vi "RemoteForOldJoystick.vi"() -> ()   [LabVIEW 2020]
uses:
  oldStudicaJoystick.ctl
  <vilib>/Platform/TimedLoop/XDataNode/timing_clust.ctl
  <vilib>/Platform/TimedLoop/XDataNode/nitl_modes.ctl
  <vilib>/Platform/TimedLoop/XDataNode/wakeup.ctl
  <vilib>/CISH Robotics/L4VMX TitanQuad/Motor ID.ctl
  <vilib>/CISH Robotics/L4VMX VMXpi/Type Def/VMX Channel Index.ctl
  <vilib>/CISH Robotics/L4VMX TitanQuad/TitanQuad.lvclass
  <vilib>/platform/TimedLoop/XDataNode/XDataNode.xnode
  <vilib>/ReMiSYS Technology/RemoteToolkit/Receiver/Receiver.lvclass
  <vilib>/CISH Robotics/L4VMX VMXpi/L4VMX.lvlib
  <vilib>/CISH Robotics/L4VMX VMXpi/Digital Input/Digital Input.lvclass
  <vilib>/Platform/TimedLoop/XDataNode/XDNodeRunTimeDep.lvlib
panel:
  in  "turnSpeed":dbl=100.0
  in  "reset Encoder":bool
  out "Finished Late? [i-1]":bool
  in  "error in (no error)":errorcluster
  out "Enc [M0, M1, M2] (deg)":dbl[](array[numeric])
  out "error out":errorcluster
  out "StudicaJoystick":T1
  out "Stop0":bool
  out "Error Out":errorcluster
  in  "Stop":bool
  out "Received?":bool
  # "61 * 16"
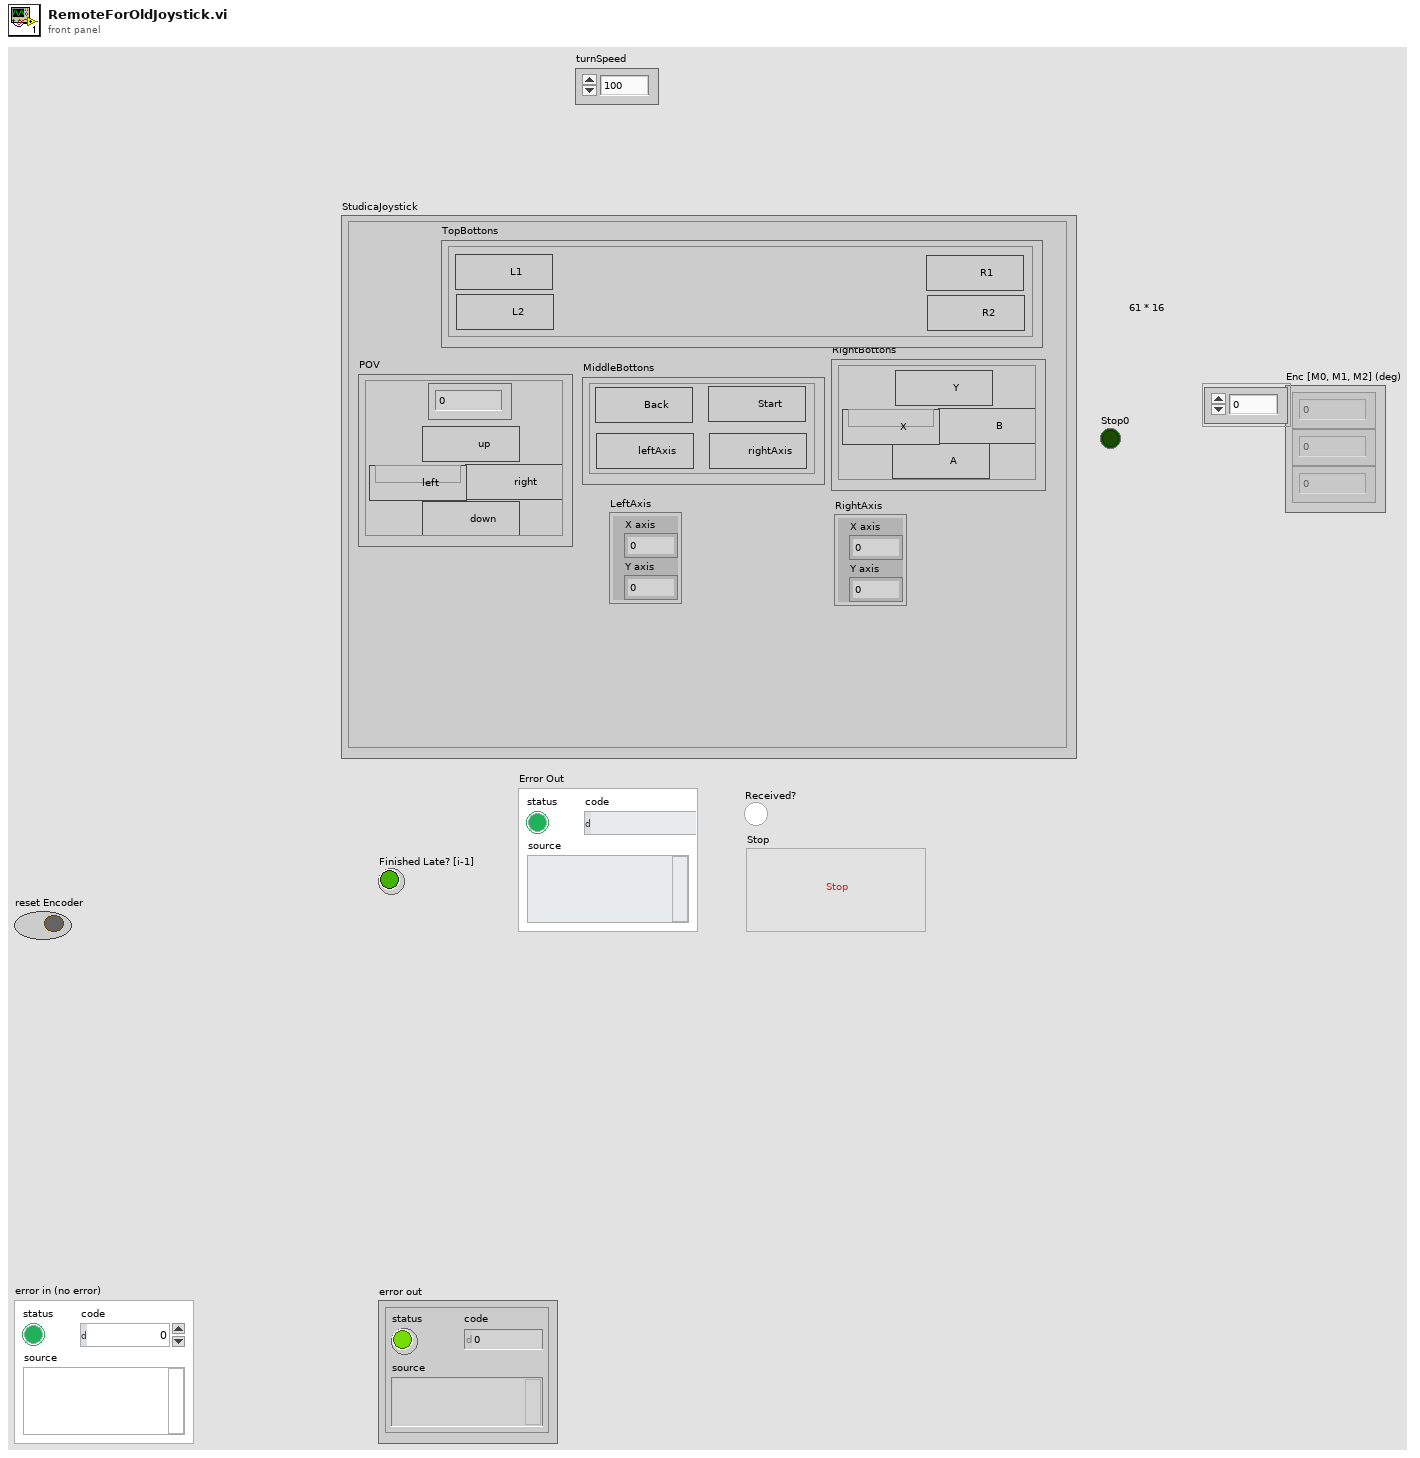
[diagram p1: front panel]
types:
  T1 = typedef "oldStudicaJoystick.ctl" = cluster{"LeftAxis":cluster{"X axis":i32, "Y axis":i32}, "RightAxis":cluster{"X axis":i32, "Y axis":i32}, "RightBottons":cluster{"A":bool, "B":bool, "X":bool, "Y":bool}, "TopBottons":cluster{"Left1":bool, "Left2":bool, "Right1":bool, "Right2":bool}, "MiddleBottons":cluster{"Back":bool, "Play Button":bool, "leftAxis":bool, "rightAxis":bool}, "POV":cluster{"right":bool, "left":bool, "up":bool, "direction":i32, "down":bool}}
  T2 = typedef "TitanQuad.lvlib/TitanQuad.lvclass/Motor ID.ctl" = enum16{"M0", "M1", "M2", "M3"}
  T3 = typedef "XDNodeRunTimeDep.lvlib/timing_clust.ctl" = cluster{"Expected End [f-1]":u64, "Actual End [f-1]":u64, "Finished Late? [f-1]":bool, "Expected End [i-1]":u64, "Actual End [i-1]":u64, "Finished Late? [i-1]":bool, "Expected Start [i]":u64, "Actual Start [i]":u64, "Expected Start [f]":u64, "Actual Start [f]":u64, "Source Name":string, "Structure Name":string, "Period":i64, "Deadline":i64, "Offset":i64, "Start":i64, "Priority":i32, "Timeout":i32, "Mode":T4, "Wakeup Reason":T5, "Error":errorcluster, "Source Type":string, "Secondary Source Type":string, "Global End Time":u64, "Global Start Time":u64, "Frame Duration":u64, "Iteration Duration":u64, "Assigned CPU":i32, "I/O Scan Engine Mode":u32}
  T4 = typedef "XDNodeRunTimeDep.lvlib/nitl_modes.ctl" = enum32{"No Change", "Process missed periods, maintain original phase", "Discard missed periods, maintain original phase", "Process missed periods, ignore original phase", "Discard missed periods, ignore original phase"}
  T5 = typedef "XDNodeRunTimeDep.lvlib/wakeup.ctl" = enum32{"Normal", "Aborted", "Asynchronous wakeup", "Timing source error", "Timed loop error", "Timeout"}
  T6 = typedef "L4VMX.lvlib/VMX Channel Index.ctl" = enum16{"0", "1", "2", "3", "4", "5", "6", "7", "8", "9", "10", "11", "12", "13", "14", "15", "16", "17", "18", "19", "20", "21", "22", "23", "24", "25", "26", "27", "28", "29", "30", "31", "32", "33"}
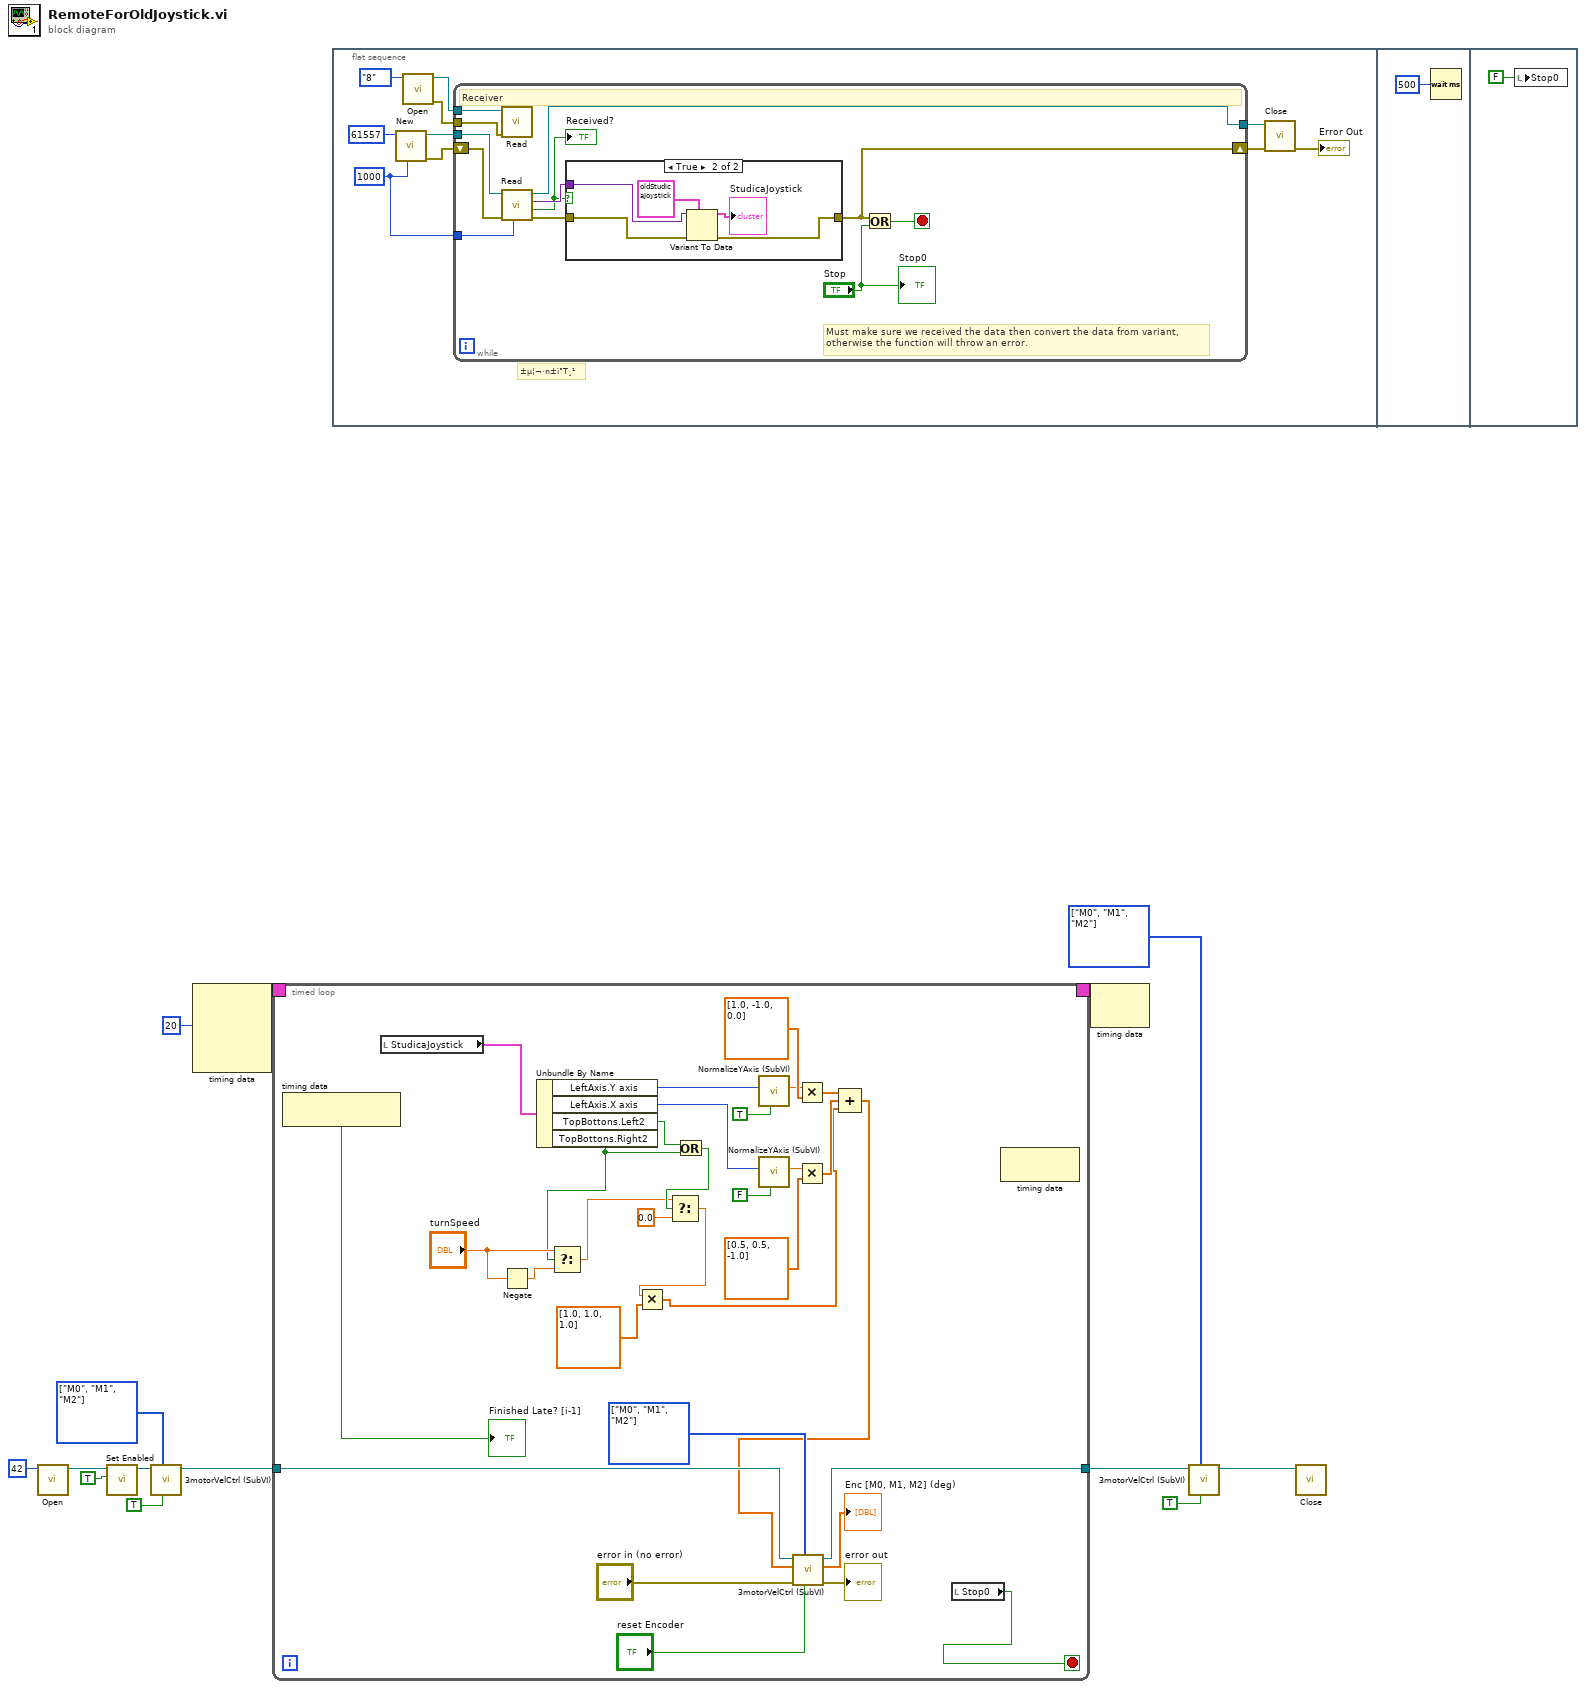
[diagram p0: block diagram]
diagram:
  w3 = T2[] [enum."M0", enum."M1", enum."M2"] items=["M0", "M1", "M2", "M3"] ("motorPort [M0, M1, M2]")
  w4 = T2[] [enum."M0", enum."M1", enum."M2"] items=["M0", "M1", "M2", "M3"] ("motorPort [M0, M1, M2]")
  n1 = call <vilib>:"Open.vi"("Titan ID (42)"=u8 42) -> ("TitanQuad Object"=w12:refnum<class "TitanQuad.lvclass">)  [unwired: 9 in, 1 out]
  n2 = call <vilib>:"Set Enabled.vi"("Enable"=TRUE, "TitanQuad Object"=w12) -> ("TitanQuad Object"=w6:refnum<class "TitanQuad.lvclass">)  [unwired: 8 in, 1 out]
  n3 = call "3motorVelCtrl (SubVI).vi"("reset Encoder"=TRUE, "motorPort [M0, M1, M2]"=w4, "TitanQuad in"=w6) -> ("TitanQuad out"=w5:refnum<class "TitanQuad.lvclass">)  [unwired: 6 in, 2 out]
  n4 = node-c288(i64 20 ("Period")) -> (w14:T3)  [unwired: 3 in]
  n5 = timed-loop {
    tunnel: w5 -> [w43]
    tunnel: [w45] -> w8
    timing: w14 -> [_]
    timing-out: [_] -> w13
    stop <- w15 stop-if-true
    w38 = T2[] [enum."M0", enum."M1", enum."M2"] items=["M0", "M1", "M2", "M3"] ("motorPort [M0, M1, M2]")
    n6 = node-c288() -> (→"Finished Late? [i-1]":bool)  [unwired: 1 in]
    n7 = local read "StudicaJoystick"() -> (w27:T1)
    n8 = Negate(x="turnSpeed") -> (-x=w26:dbl)
    n9 = Unbundle By Name(w27) -> ("LeftAxis.Y axis"=w28:i32, "LeftAxis.X axis"=w30:i32, "TopBottons.Left2"=w21:bool, "TopBottons.Right2"=w20:bool)
    n10 = Select(t="turnSpeed", s=w20, f=w26) -> (s? t:f=w18:dbl)
    n11 = Or(x=w21, y=w20) -> (x .or. y?=w19:bool)
    n12 = Select(t=w18, s=w19, f=0.0) -> (s? t:f=w16:dbl)
    n13 = Multiply(x=w16, y=dbl[] [1.0, 1.0, 1.0]) -> (x*y=w23:dbl[])
    n14 = call "NormalizeYAxis (SubVI).vi"("negative?"=TRUE, "Yaxis"=w28) -> ("NormalizedAxis"=w32:dbl)  [unwired: 9 in]
    n15 = call "NormalizeYAxis (SubVI).vi"("negative?"=FALSE, "Yaxis"=w30) -> ("NormalizedAxis"=w35:dbl)  [unwired: 9 in]
    n16 = Multiply(x=w32, y=dbl[] [1.0, -1.0, 0.0]) -> (x*y=w36:dbl[])
    n17 = Multiply(x=w35, y=dbl[] [0.5, 0.5, -1.0]) -> (x*y=w37:dbl[])
    n18 = Compound Arithmetic op=ADD(w36, w37, w23) -> (w22:dbl[])
    n19 = call "3motorVelCtrl (SubVI).vi"("reset Encoder"="reset Encoder", "motorPort [M0, M1, M2]"=w38, "error in (no error)"="error in (no error)", "motorSpeed [M0, M1, M2] (deg/s)"=w22, "TitanQuad in"=w43) -> ("error out"=→"error out":errorcluster, "Enc [M0, M1, M2] (deg)"=→"Enc [M0, M1, M2] (deg)":dbl[], "TitanQuad out"=w45:refnum<class "TitanQuad.lvclass">)  [unwired: 4 in]
    n20 = local read "Stop0"() -> (w15:bool)
    n21 = node-c288() -> ()  [unwired: 1 in, 1 out]
  }
  n22 = flat-sequence {
    frame #0 {
      w54 = 1000 ("Timeout ms (25000)")
      # "±µ¦¬·n±ì°T¸¹"
      n23 = call <vilib>:"New.vi"("Timeout ms (25000)"=w54, "Port (61557)"=u16 61557) -> ("Error Out"=w58:errorcluster, "Receiver Ref."=w57:refnum<class "Receiver.lvclass">)  [unwired: 8 in]
      n24 = call <vilib>:"Open.vi"("VMX Channel Index"=VMX_Channel_Index."8") -> ("Error Out"=w49:errorcluster, "Digital Input Object"=w50:refnum<class "Digital Input.lvclass">)  [unwired: 9 in]
      n25 = while {
        shift-right: [w63] -> w56
        shift-left: w58 -> [w70]
        tunnel: w57 -> [w69]
        tunnel: [w68] -> w55
        tunnel: w54 -> [w67]
        tunnel: w50 -> [w61]
        tunnel: w49 -> [w60]
        stop <- w66 stop-if-true
        # "Must make sure we received the data then convert the data from variant,\notherwise the function will throw an error."
        # "Receiver"
        n26 = call <vilib>:"Read.vi"("Error In"=w60, "Digital Input Object"=w61) -> ()  [unwired: 7 in, 3 out]
        n27 = call <vilib>:"Read.vi"("Timeout ms (1000)"=w67, "Error In"=w70, "Receiver Ref."=w69) -> ("Error Out"=w65:errorcluster, "Received?"=w62:bool, "Value"=w64:variant, "Receiver Ref."=w68:refnum<class "Receiver.lvclass">)  [unwired: 5 in]
        "Received?" <- w62
        n28 = case shown="True" w62 {
          tunnel: w65 -> [w71 w76]
          tunnel: w64 -> [_ w75]
          tunnel: [w71 w74] -> w63
          frame False {
          }
          frame True {
            n29 = Variant To Data(error in=w76, type=T1 {"LeftAxis"={"X axis"=0, "Y axis"=0}, "RightAxis"={"X axis"=0, "Y axis"=0}, "RightBottons"={"A"=FALSE, "B"=FALSE, "X"=FALSE, "Y"=FALSE}, "TopBottons"={"Left1"=FALSE, "Left2"=FALSE, "Right1"=FALSE, "Right2"=FALSE}, "MiddleBottons"={"Back"=FALSE, "Play Button"=FALSE, "leftAxis"=FALSE, "rightAxis"=FALSE}, "POV"={"right"=FALSE, "left"=FALSE, "up"=FALSE, "direction"=0, "down"=FALSE}} ("OldStudicaJoystick"), Variant=w75) -> (data=→"StudicaJoystick":T1, error out=w74:errorcluster)
          }
        }
        n30 = Or(x=w63, y="Stop") -> (x .or. y?=w66:bool)
        "Stop0" <- "Stop"
      }
      n31 = call <vilib>:"Close.vi"("Error In"=w56, "Receiver Ref."=w55) -> ("Error Out"=→"Error Out":errorcluster)  [unwired: 9 in]
    }
    frame #1 {
      n32 = Wait (ms)(milliseconds to wait=u32 500) -> ()  [unwired: 1 out]
    }
    frame #2 {
      n33 = local write "Stop0"(FALSE ("Stop")) -> ()
    }
  }
  n34 = node-c288(w13) -> ()  [unwired: 1 out]
  n35 = call "3motorVelCtrl (SubVI).vi"("reset Encoder"=TRUE, "motorPort [M0, M1, M2]"=w3, "TitanQuad in"=w8) -> ("TitanQuad out"=w2:refnum<class "TitanQuad.lvclass">)  [unwired: 6 in, 2 out]
  n36 = call <vilib>:"Close.vi"("TitanQuad Object"=w2) -> ()  [unwired: 10 in, 1 out]
